vi "SetDigitalPosition.vi"(8 "Position":i32, 10 "Controller Channel":i64, 11 "Handle":u64) -> (3 "FT_Status":u64(ring) items=["FT_OK", "FT_INVALID_HANDLE", "FT_DEVICE_NOT_FOUND", "FT_DEVICE_NOT_OPENED", "FT_IO_ERROR", "FT_INSUFFICIENT_RESOURCES", "FT_INVALID_PARAMETER", "FT_INVALID_BAUD_RATE", "FT_DEVICE_NOT_OPENED_FOR_ERASE", "FT_DEVICE_NOT_OPENED_FOR_WRITE", "FT_FAILED_TO_WRITE_DEVICE", "FT_EEPROM_READ_FAILED", "FT_EEPROM_WRITE_FAILED", "FT_EEPROM_ERASE_FAILED", "FT_EEPROM_NOT_PRESENT", "FT_EEPROM_NOT_PROGRAMMED", "FT_INVALID_ARGS", "FT_NOT_SUPPORTED", "FT_OTHER_ERROR"])   [LabVIEW 2018]
panel:
  out "Bytes Written":u64
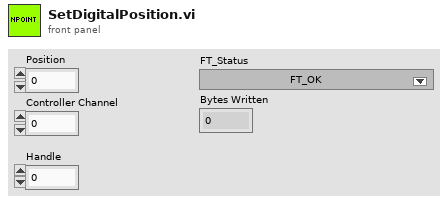
[diagram p1: front panel]
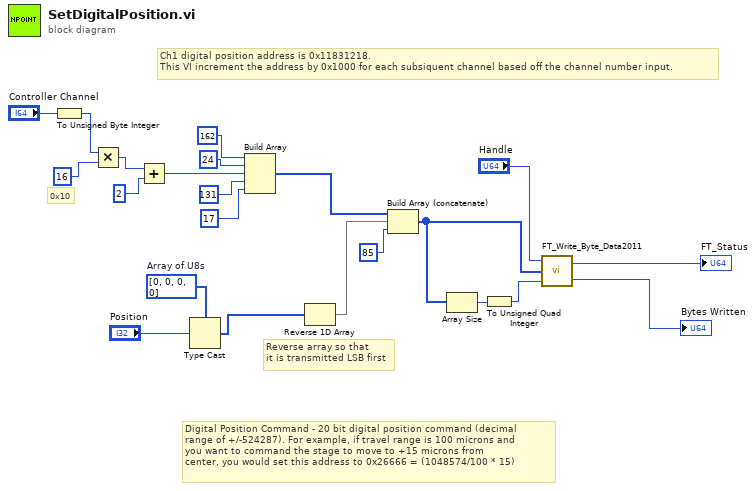
[diagram p0: block diagram]
diagram:
  w16 = u8[] [0, 0, 0, 0]  # Array of U8s
  # "Digital Position Command - 20 bit digital position command (decimal\nrange of +/-524287). For example, if travel range is 100 microns and\nyou want to command the stage to move to +15 microns from\ncenter, you would set this address to 0x26666 = (1048574/100 * 15)"
  # "Ch1 digital position address is 0x11831218.\nThis VI increment the address by 0x1000 for each subsiquent channel based off the channel number input."
  # "Reverse array so that\nit is transmitted LSB first"
  # "0x10"
  n1 = To Unsigned Byte Integer(number="Controller Channel") -> (unsigned 8bit integer=w1:u8)
  n2 = Multiply(x=w1, y=u8 16) -> (x*y=w4:u8)
  n3 = Add(x=w4, y=u8 2 ("element")) -> (x+y=w3:u8)
  n4 = Type Cast(type=w16, x="Position") -> (*(type *) &x=w12:u8[])
  n5 = Build Array(u8 162 ("element"), u8 24 ("element"), w3, u8 131 ("element"), u8 17 ("element")) -> (w15:u8[])
  n6 = Reverse 1D Array(array=w12) -> (reversed array=w11:u8[])
  n7 = Build Array (concatenate)(w15, w11, u8 85 ("element")) -> (w13:u8[])
  n8 = Array Size(array=w13) -> (size(s)=w22:i32)
  n9 = To Unsigned Quad Integer(1:w22) -> (0:w21:u64)
  n10 = call "FT_Write_Byte_Data2011.vi"("Bytes To Write"=w21, "Buffer"=w13, "Handle"="Handle") -> ("Bytes Written"=→"Bytes Written":u64, "FT_Status"=→"FT_Status":u64)
